vi "Unflatten to PDU.vi"(8 "error in (no error)":errorcluster, 10 "Modbus data unit data":u8[](array[numeric])) -> (0 "error out":errorcluster, 3 "Modbus data unit out":refnum<class "Modbus Data Unit (PDU).lvclass">)   [LabVIEW 2020, in "SubVIs.lvlib" / "Modbus Data Unit (PDU).lvclass"]
uses:
  <vilib>/Modbus/subvis/Modbus Data Unit (PDU)/Modbus Data Unit (PDU).lvclass
  <vilib>/Modbus/subvis/Modbus Data Unit (PDU)/Modbus Data Unit (PDU).lvclass/Modbus Data Unit (PDU).ctl
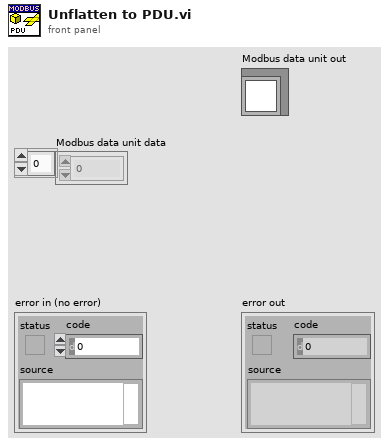
[diagram p1: front panel]
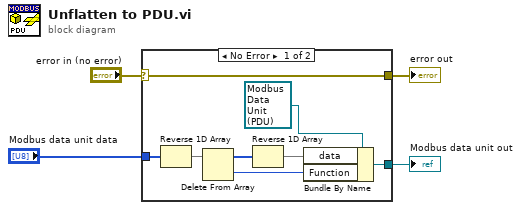
[diagram p0: block diagram]
diagram:
  n1 = case shown="No Error" "error in (no error)" {
    selector: "error in (no error)" -> [w5 w13]
    tunnel: [w12 _] -> w4
    tunnel: "Modbus data unit data" -> [w9 _]
    tunnel: [w5 w13] -> w1
    frame No Error {
      n2 = Reverse 1D Array(array=w9) -> (reversed array=w8:u8[])
      n3 = Delete From Array(array=w8) -> (deleted portion=w10:u8, array with subset deleted=w6:u8[])  [unwired: 2 in]
      n4 = Reverse 1D Array(array=w6) -> (reversed array=w7:u8[])
      n5 = Bundle By Name(cluster=refnum<class "Modbus Data Unit (PDU).lvclass"> refnum ("modbus data unit"), "data"=w7, "Function"=w10) -> (w12:refnum<class "Modbus Data Unit (PDU).lvclass">)
    }
    frame Error {
    }
  }
  "error out" <- w1
  "Modbus data unit out" <- w4
